vi "NewVSS_GoTo.vi"(6 "VSSStates":T1, 7 "Numeric":i32, 8 "Path  Smooth":dbl[][](array[numeric]), 9 "Position":dbl[](array[numeric]), 10 "V_tan(opitional)":dbl, 11 "GoToNavigation?":bool=TRUE) -> (3 "Output Velocity":dbl[](array[numeric]) format="%.2f")   [LabVIEW 2023]
uses:
  VSSAttackerStates.ctl
  Utilities_class/Utilities.lvclass
  <vilib>/Analysis/coordinate.llb/2D Cartesian Coordinate Rotation (Scalar).vi
  <vilib>/Analysis/NI_AALPro.lvlib
panel:
  in  "Limits":cluster{"output high":dbl, "output low":dbl}={"output high"=4.0, "output low"=-4.0}
  in  "PID gains in":T2={"proportional gain (Kc)"=1.5, "integral time (Ti, min)"=0.0, "derivative time (Td, min)"=10.0}
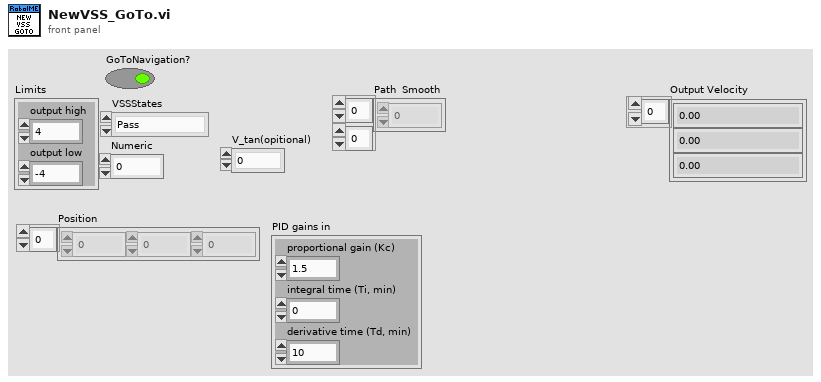
[diagram p1: front panel]
types:
  T1 = typedef "VSSAttackerStates.ctl" = enum16{"Pass", "GoToTangent", "BallGetting", "GoToKick", "Rotate anti-clockwise", "Rotate Clockwise", ""}
  T2 = cluster{"proportional gain (Kc)":dbl, "integral time (Ti, min)":dbl, "derivative time (Td, min)":dbl}
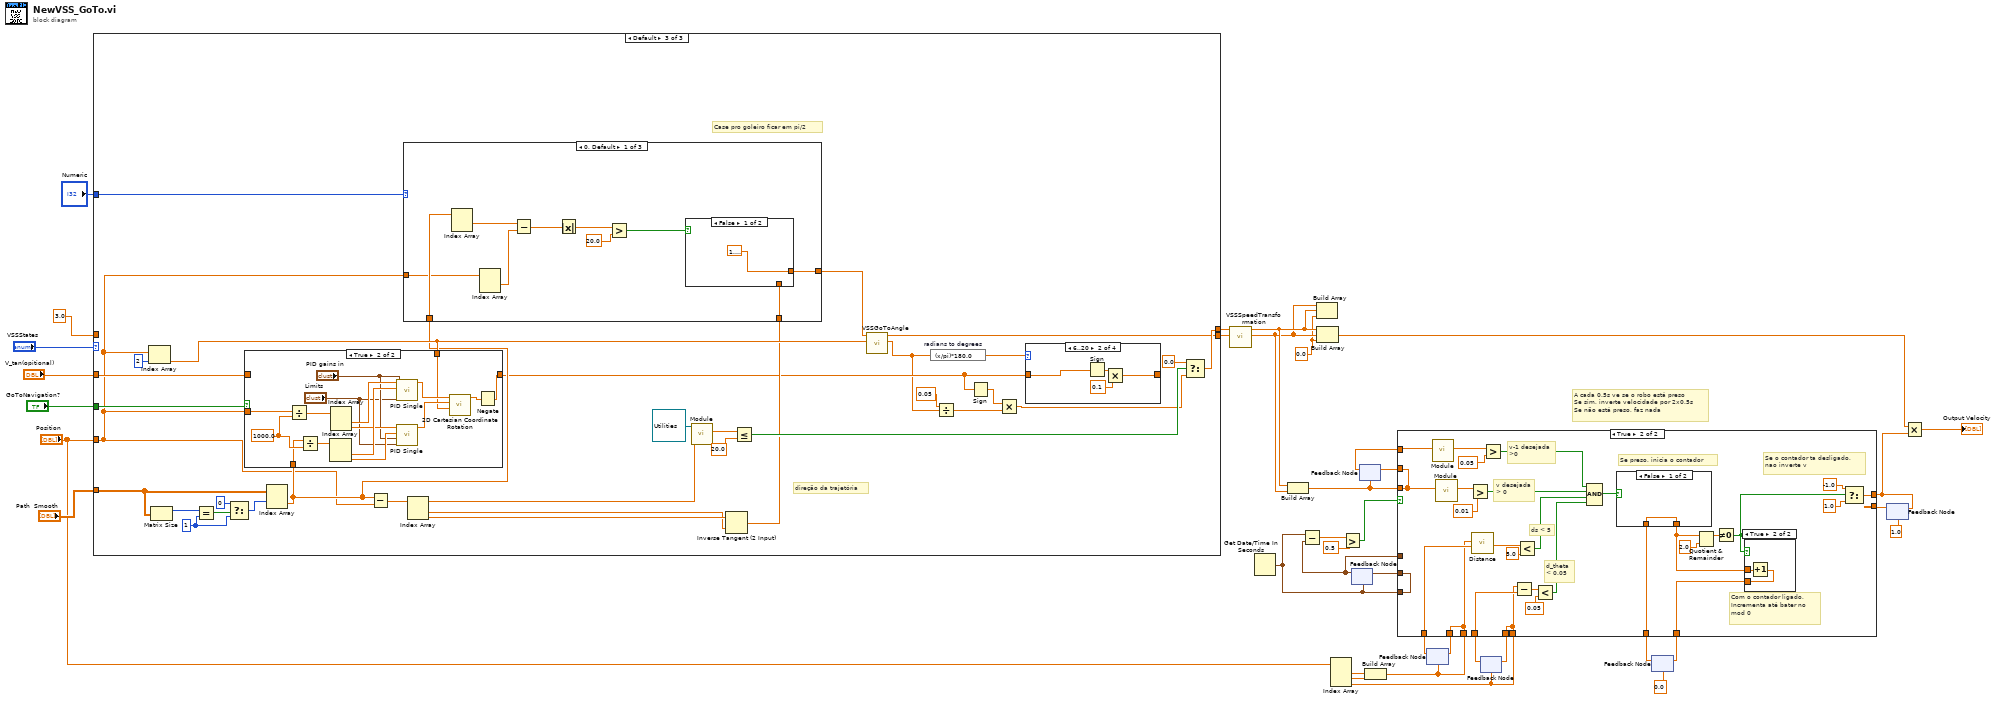
[diagram p0: block diagram]
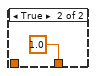
[diagram p4: hidden frame]
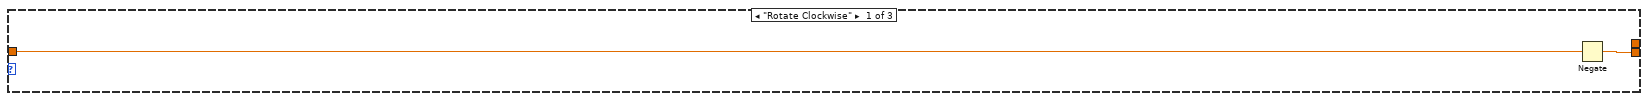
[diagram p5: hidden frame]
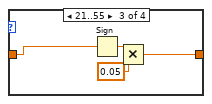
[diagram p12: hidden frame]
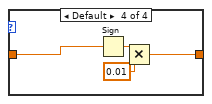
[diagram p13: hidden frame]
diagram:
  w5 = 0.0 ("element")
  # "A cada 0.5s ve se o robo está preso\nSe sim, inverte velocidade por 2x0.5s\nSe não está preso, faz nada"
  n1 = case shown="Default" "VSSStates" {
    tunnel: [w39 w40 w47] -> w37
    tunnel: "Path  Smooth" -> [_ _ w69]
    tunnel: [_ _ w57] -> w35
    tunnel: "Position" -> [_ _ w48]
    tunnel: "GoToNavigation?" -> [_ _ w54]
    tunnel: "V_tan(opitional)" -> [_ _ w53]
    tunnel: 3.0 -> [w38 w40 _]
    tunnel: "Numeric" -> [_ _ w52]
    frame "Rotate Clockwise" {
      n2 = Negate(x=w38) -> (-x=w39:dbl)
    }
    frame "Rotate anti-clockwise" {
    }
    frame Default {
      w65 = 1 ("y")
      # "Case pro goleiro ficar em pi/2"
      # "direção da trajetória"
      n3 = Index Array(array=w48, index=2) -> (element=w56:dbl)
      n4 = Matrix Size(0:w69) -> (1:w68:i32)  [unwired: 1 out]
      n5 = Equal?(x=w68, y=w65) -> (x = y?=w67:bool)
      n6 = Select(t=0, s=w67, f=w65) -> (s? t:f=w64:i32)
      n7 = Index Array(array=w69, index (row)=w64) -> (element=w51:dbl[])  [unwired: 1 in]
      n8 = case shown="True" w54 {
        tunnel: w51 -> [_ w91]
        tunnel: w48 -> [_ w90]
        tunnel: w56 -> [_ w89]
        tunnel: [w87 w88] -> w46
        tunnel: w53 -> [w87 _]
        frame False {
        }
        frame True {
          w92 = 1000.0
          n9 = Divide(x=w90, y=w92) -> (x/y=w94:dbl[])
          n10 = Divide(x=w91, y=w92) -> (x/y=w93:dbl[])
          n11 = Index Array(array=w93) -> (element #1=w102:dbl, element #2=w100:dbl)  [unwired: 2 in]
          n12 = Index Array(array=w94) -> (element #1=w103:dbl, element #2=w101:dbl)  [unwired: 2 in]
          n13 = call "PID Single.vi"("Limits"="Limits", "PID gains in"="PID gains in", "Variable"=w102, "Setpoint"=w103) -> ("Out"=w97:dbl)  [unwired: 7 in]
          n14 = call "PID Single.vi"("Limits"="Limits", "PID gains in"="PID gains in", "Variable"=w100, "Setpoint"=w101) -> ("Out"=w96:dbl)  [unwired: 7 in]
          n15 = call-poly <vilib>:"2D Cartesian Coordinate Rotation.vi"("theta"=w89, "y"=w96, "x"=w97) -> ("x out"=w95:dbl)  [unwired: 6 in, 2 out]
          n16 = Negate(x=w95) -> (-x=w88:dbl)
        }
      }
      n17 = Subtract(x=w51, y=w48) -> (x-y=w63:dbl[])
      n18 = Index Array(array=w63) -> (element #1=w70:dbl, element #2=w71:dbl)  [unwired: 2 in]
      n19 = call "Module.vi"("2D vector"=w63, "Utilities in"=refnum<class "Utilities.lvclass"> refnum) -> ("Modulo"=w61:dbl)  [unwired: 7 in, 2 out]
      n20 = Inverse Tangent (2 Input)(1:w70, 2:w71) -> (0:w50:dbl)
      n21 = case shown="0, Default" w52 {
        tunnel: w51 -> [w82 _ _]
        tunnel: w48 -> [w80 _ _]
        tunnel: w50 -> [w74 w85 w86]
        tunnel: [w73 w85 w86] -> w49
        frame 0, Default {
          n22 = Index Array(array=w82) -> (element #1=w79:dbl)  [unwired: 2 in, 1 out]
          n23 = Index Array(array=w80) -> (element #1=w78:dbl)  [unwired: 2 in, 1 out]
          n24 = Subtract(x=w79, y=w78) -> (x-y=w77:dbl)
          n25 = Absolute Value(x=w77) -> (abs(x)=w75:dbl)
          n26 = Greater?(x=w75, y=20.0) -> (0:w81:bool)
          n27 = case shown="False" w81 {
            tunnel: w74 -> [_ w84]
            tunnel: [1.5707963267948966 w84] -> w73
            frame False {
            }
            frame True {
            }
          }
        }
        frame 1 {
        }
        frame 2 {
        }
      }
      n28 = Less Or Equal?(x=w61, y=20.0) -> (x <= y?=w59:bool)
      n29 = call "VSSGoToAngle.vi"("orientation"=w56, "dest_orientation"=w49) -> ("AngleError"=w43:dbl, "v_ang"=w47:dbl)  [unwired: 7 in, 1 out]
      n30 = expression code="(x/pi)*180.0" "radians to degrees"(w43) -> (w72:dbl)
      n31 = Divide(x=0.05, y=w43) -> (x/y=w42:dbl)
      n32 = Sign(1:w46) -> (0:w45:dbl)
      n33 = Multiply(x=w45, y=w42) -> (x*y=w44:dbl)
      n34 = case shown="6..20" w72 {
        tunnel: w46 -> [w104 w108 w109 w116]
        tunnel: [w104 w106 w110 w114] -> _
        frame 0..5 {
        }
        frame 6..20 {
          n35 = Sign(1:w108) -> (0:w107:dbl)
          n36 = Multiply(x=w107, y=0.1) -> (x*y=w106:dbl)
        }
        frame 21..55 {
          n37 = Sign(1:w109) -> (0:w112:dbl)
          n38 = Multiply(x=w112, y=0.05) -> (x*y=w110:dbl)
        }
        frame Default {
          n39 = Sign(1:w116) -> (0:w115:dbl)
          n40 = Multiply(x=w115, y=0.01) -> (x*y=w114:dbl)
        }
      }
      n41 = Select(t=0.0, s=w59, f=w44) -> (s? t:f=w57:dbl)
    }
  }
  n42 = call "VSSSpeedTransformation.vi"("V_ang in"=w37, "V_tang in"=w35) -> ("V_rigth"=w6:dbl, "V_left"=w7:dbl)  [unwired: 8 in]
  n43 = Get Date/Time In Seconds() -> (seconds since 1Jan1904=w25:timestamp)
  n44 = Build Array(w7, w6) -> (w15:dbl[])
  n45 = Build Array(w6, w7, w5) -> ()  [unwired: 1 out]
  n46 = Build Array(w7, w6, w5) -> (w28:dbl[])
  n47 = Index Array(array="Position") -> (element #1=w11:dbl, element #2=w10:dbl, element #3=w8:dbl)  [unwired: 3 in]
  n48 = feedback #1(w25) -> (w26:timestamp)
  n49 = Subtract(x=w25, y=w26) -> (x-y=w23:dbl)
  n50 = Greater?(x=w23, y=0.5) -> (0:w20:bool)
  n51 = feedback #2(w15) -> (w14:dbl[])
  n52 = Build Array(w11, w10) -> (w9:dbl[])
  n53 = feedback #3(w9) -> (w29:dbl[])
  n54 = feedback #4(w8) -> (w21:dbl)
  n55 = feedback #5(0.0 ("element")) -> (w1:dbl)
  n56 = feedback #6(1.0 ("element")) -> (w19:dbl)
  n57 = case shown="True" w20 {
    tunnel: w15 -> [_ w131]
    tunnel: w29 -> [w121 w151]
    tunnel: w9 -> [_ w139]
    tunnel: w26 -> [w122 _]
    tunnel: w25 -> [_ w140]
    tunnel: [w122 w140] -> w24
    tunnel: w21 -> [w120 w142]
    tunnel: w8 -> [_ w138]
    tunnel: [w118 w123] -> w4
    tunnel: w19 -> [w118 _]
    tunnel: [w121 w139] -> w17
    tunnel: [w120 w138] -> w16
    tunnel: w14 -> [w119 w134]
    tunnel: [w119 w131] -> w13
    tunnel: [w117 w126] -> w2
    tunnel: w1 -> [w117 w129]
    frame False {
    }
    frame True {
      # "Se o contador ta desligado,\nnao inverte v"
      # "Com o contador ligado,\nIncrementa até bater no \nmod 0"
      # "Se preso, inicia o contador"
      # "v-1 desejada\n>0"
      # "v desejada\n> 0"
      # "ds < 5"
      # "d_theta \n< 0.05"
      n58 = call "Module.vi"("2D vector"=w134) -> ("Modulo"=w133:dbl)  [unwired: 8 in, 2 out]
      n59 = call "Module.vi"("2D vector"=w131) -> ("Modulo"=w150:dbl)  [unwired: 8 in, 2 out]
      n60 = Greater?(x=w150, y=0.01) -> (0:w146:bool)
      n61 = call "Distance.vi"("P1"=w151, "P2"=w139) -> ("Distance"=w148:dbl)  [unwired: 7 in, 2 out]
      n62 = Greater?(x=w133, y=0.05) -> (0:w132:bool)
      n63 = Subtract(x=w138, y=w142) -> (x-y=w143:dbl)
      n64 = Less?(x=w148, y=5.0) -> (x < y?=w137:bool)
      n65 = Less?(x=w143, y=0.05) -> (x < y?=w136:bool)
      n66 = Compound Arithmetic op=AND(w132, w146, w137, w136) -> (w130:bool)
      n67 = case shown="False" w130 {
        tunnel: [w155 1.0 ("element")] -> w127
        tunnel: w129 -> [w155 _]
        frame False {
        }
        frame True {
        }
      }
      n68 = Quotient & Remainder(x=w127, y=2.0 ("element")) -> (x-y*floor(x/y)=w125:dbl)  [unwired: 1 out]
      n69 = Not Equal To 0?(x=w125) -> (x != 0?=w124:bool)
      n70 = case shown="True" w124 {
        tunnel: w127 -> [w152 w154]
        tunnel: [w152 w153] -> w126
        frame False {
        }
        frame True {
          n71 = Increment(x=w154) -> (x+1=w153:dbl)
        }
      }
      n72 = Select(t=-1.0 ("element"), s=w124, f=1.0 ("element")) -> (s? t:f=w123:dbl)
    }
  }
  n73 = feedback-in #1(w24) -> ()
  n74 = feedback-in #2(w13) -> ()
  n75 = feedback-in #3(w17) -> ()
  n76 = feedback-in #4(w16) -> ()
  n77 = feedback-in #5(w2) -> ()
  n78 = feedback-in #6(w4) -> ()
  n79 = Multiply(x=w28, y=w4) -> (x*y=→"Output Velocity":dbl[])
